vi "Draw Grid.vi"(8 "error in (no error)":errorcluster, 9 "color":u32(colorbox)=16777238, 11 "dialog info in":T1={"steering frame ref"=refnum, "active wheel indexes"=[], "FP Refs"={"VI Refnum"=refnum, "Menu Ref"=refnum, "Sub Panel"=refnum, "picture"=refnum, "Steering Type"=refnum, "zoom in"=refnum, "zoom out"=refnum, "zoom extents"=refnum, "Wheels"=refnum, "Add Wheel"=refnum, "Remove Wheel"=refnum, "Copy Wheel"=refnum, "Angle Units"=refnum}, "subpanel info"={"subpanel VI refs"=[], "subpanel types"=[], "main to subpanel command events"=[]}, "picture dragging state"={"dragging"=FALSE, "wheel index"=-1, "dragging mode"=enum."translate", "wheel start position"={"x"=0.0, "y"=0.0, "theta"=0.0}, "relative mouse position"={"x"=0.0, "y"=0.0}, "relative mouse init angle (rad)"=0.0}, "picture size (pixels)"={"Width"=500, "Height"=500}, "picture grid"=bytes[0], "click zones group"={"click zones array"=[], "num click zones"=0}, "draw options"={"draw wheel states?"=FALSE, "highlight wheel index"=-1, "pixels per unit"=10.0, "draw forward velocity?"=FALSE, "velocity scale"=1.0}}) -> (0 "error out":errorcluster, 3 "dialog info out":T1={"steering frame ref"=refnum, "active wheel indexes"=[], "FP Refs"={"VI Refnum"=refnum, "Menu Ref"=refnum, "Sub Panel"=refnum, "picture"=refnum, "Steering Type"=refnum, "zoom in"=refnum, "zoom out"=refnum, "zoom extents"=refnum, "Wheels"=refnum, "Add Wheel"=refnum, "Remove Wheel"=refnum, "Copy Wheel"=refnum, "Angle Units"=refnum}, "subpanel info"={"subpanel VI refs"=[], "subpanel types"=[], "main to subpanel command events"=[]}, "picture dragging state"={"dragging"=FALSE, "wheel index"=-1, "dragging mode"=enum."translate", "wheel start position"={"x"=0.0, "y"=0.0, "theta"=0.0}, "relative mouse position"={"x"=0.0, "y"=0.0}, "relative mouse init angle (rad)"=0.0}, "picture size (pixels)"={"Width"=500, "Height"=500}, "picture grid"=bytes[0], "click zones group"={"click zones array"=[], "num click zones"=0}, "draw options"={"draw wheel states?"=FALSE, "highlight wheel index"=-1, "pixels per unit"=10.0, "draw forward velocity?"=FALSE, "velocity scale"=1.0}})   [LabVIEW 2017, in "NI_Robotics_Configure Steering Frame.lvlib"]
uses:
  <vilib>/robotics/Dialog/Configure Steering Frame/NI_Robotics_Configure Steering Frame.lvlib
  <vilib>/robotics/Dialog/Configure Steering Frame/Dialog Info.ctl
  <vilib>/robotics/Steering/Steering Frame/NI_Robotics_Steering Frame.lvclass
  <vilib>/robotics/Dialog/Configure Steering Frame/FP Refs.ctl
  <vilib>/robotics/Dialog/Configure Steering Frame/Subpanel Info.ctl
  <vilib>/robotics/Dialog/Configure Steering Frame/Main to Subpanel Command Event.ctl
  <vilib>/robotics/Dialog/Configure Steering Frame/Main to Subpanel Command.ctl
  <vilib>/robotics/Dialog/Configure Steering Frame/Dragging State.ctl
  <vilib>/robotics/Dialog/Configure Steering Frame/Dragging Mode.ctl
  <vilib>/Utility/miscctls.llb/LVBoundsTypeDef.ctl
  <vilib>/robotics/Dialog/Configure Steering Frame/Click Zone.ctl
  <vilib>/robotics/Utilities/Visualization/Steering Visualization/Steering Picture/Draw Steering Frame Options.ctl
  <vilib>/robotics/Utilities/Visualization/Steering Visualization/Steering Picture/NI_Robotics_Steering Picture.lvlib
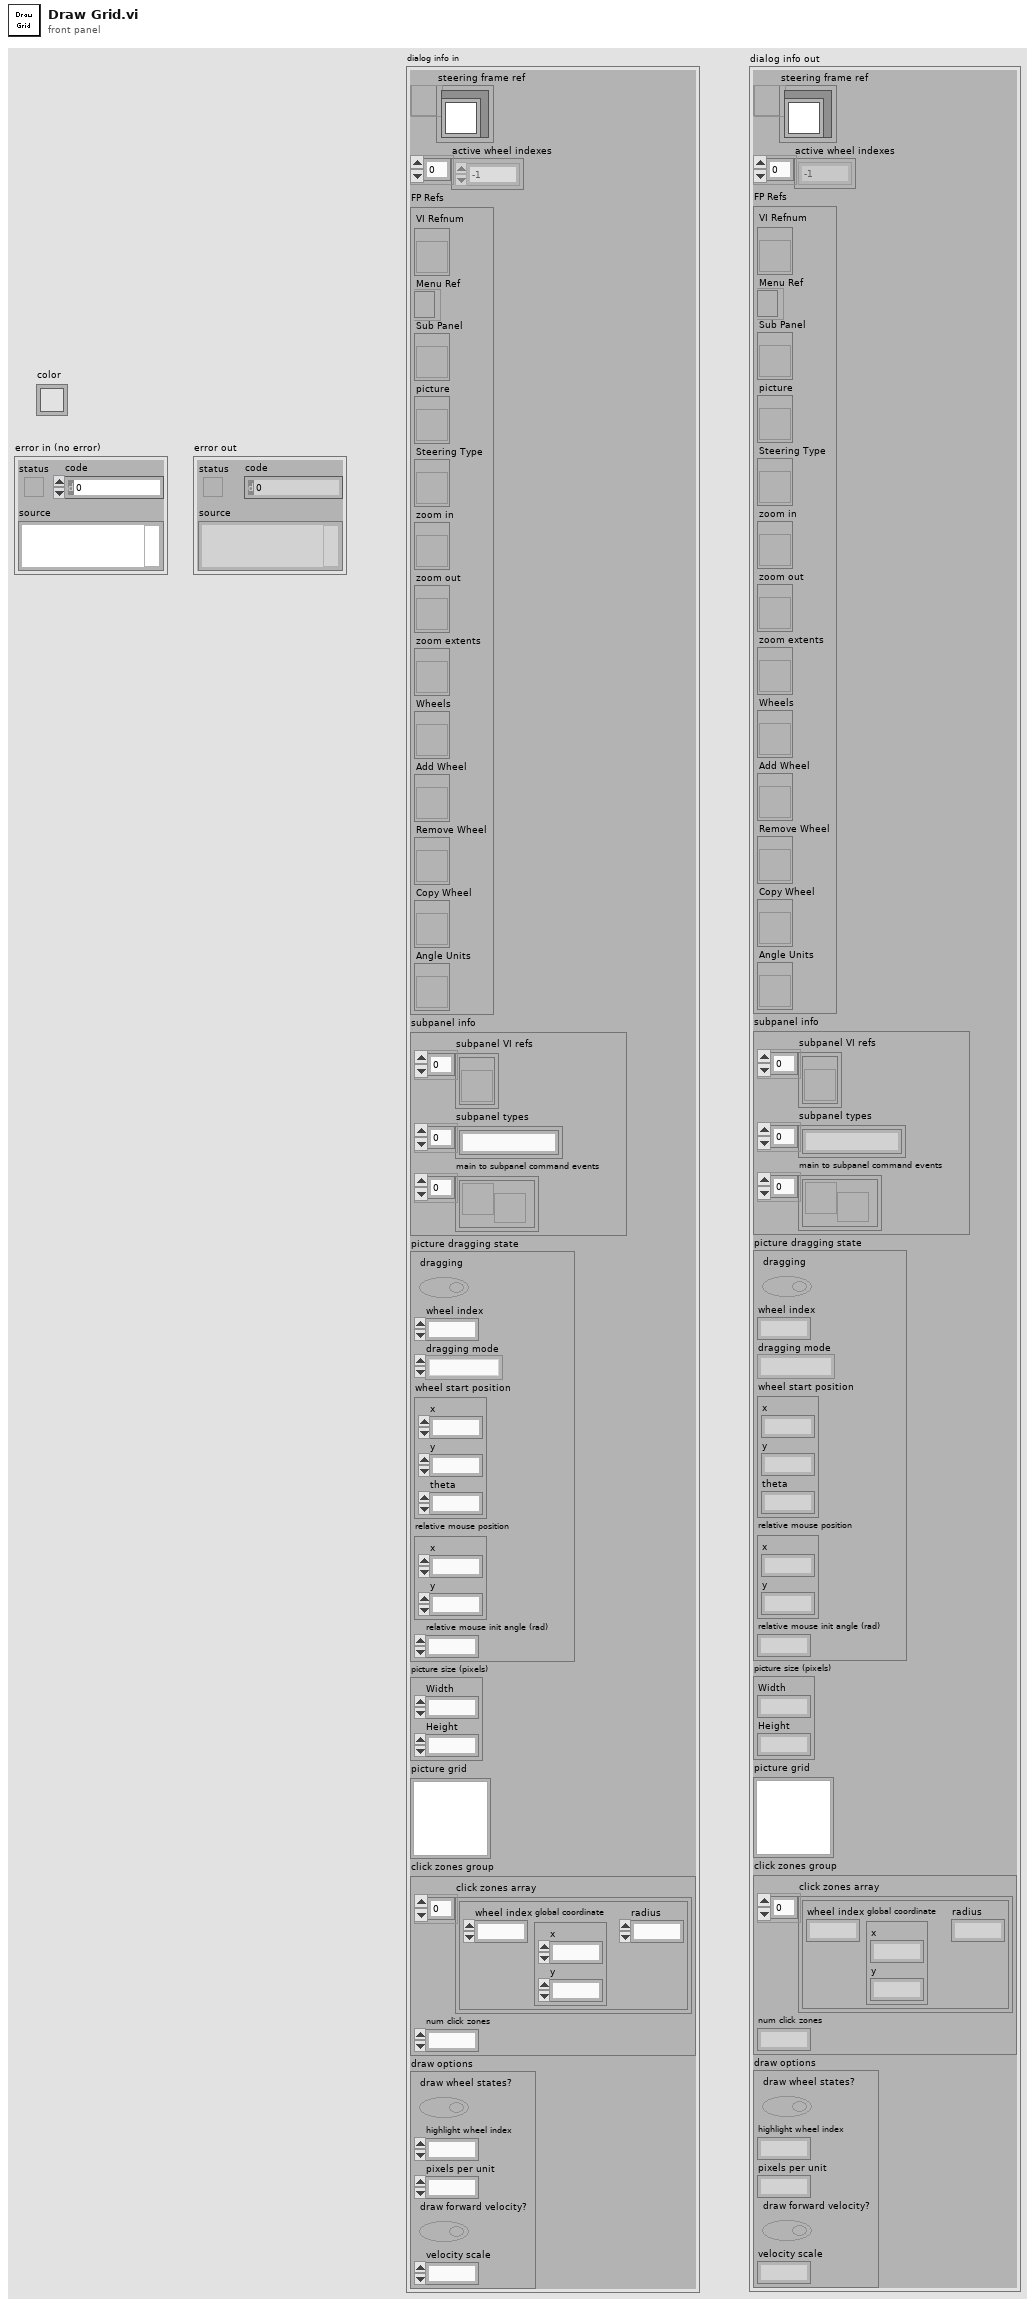
[diagram p1: front panel]
types:
  T1 = typedef "NI_Robotics_Configure Steering Frame.lvlib/Dialog Info.ctl" = cluster{"steering frame ref":refnum<data-value>, "active wheel indexes":i32[], "FP Refs":T2, "subpanel info":T3, "picture dragging state":T5, "picture size (pixels)":T7, "picture grid":picture, "click zones group":cluster{"click zones array":T8[], "num click zones":i32}, "draw options":T9}
  T2 = typedef "NI_Robotics_Configure Steering Frame.lvlib/FP Refs.ctl" = cluster{"VI Refnum":refnum<vi>, "Menu Ref":refnum<k9>, "Sub Panel":refnum<vi>, "picture":refnum<vi>, "Steering Type":refnum<vi>, "zoom in":refnum<vi>, "zoom out":refnum<vi>, "zoom extents":refnum<vi>, "Wheels":refnum<vi>, "Add Wheel":refnum<vi>, "Remove Wheel":refnum<vi>, "Copy Wheel":refnum<vi>, "Angle Units":refnum<vi>}
  T3 = typedef "NI_Robotics_Configure Steering Frame.lvlib/Subpanel Info.ctl" = cluster{"subpanel VI refs":refnum<vi>[], "subpanel types":string[], "main to subpanel command events":T4[]}
  T4 = typedef "NI_Robotics_Configure Steering Frame.lvlib/Main to Subpanel Command Event.ctl" = refnum<user-event>
  T5 = typedef "NI_Robotics_Configure Steering Frame.lvlib/Dragging State.ctl" = cluster{"dragging":bool, "wheel index":i32, "dragging mode":T6, "wheel start position":cluster{"x":dbl, "y":dbl, "theta":dbl}, "relative mouse position":cluster{"x":dbl, "y":dbl}, "relative mouse init angle (rad)":dbl}
  T6 = typedef "NI_Robotics_Configure Steering Frame.lvlib/Dragging Mode.ctl" = enum16{"translate", "rotate"}
  T7 = typedef "LVBoundsTypeDef.ctl" = cluster{"Width":u32, "Height":u32}
  T8 = typedef "NI_Robotics_Configure Steering Frame.lvlib/Click Zone.ctl" = cluster{"wheel index":i32, "global coordinate":cluster{"x":dbl, "y":dbl}, "radius":dbl}
  T9 = typedef "NI_Robotics_Steering Picture.lvlib/Draw Steering Frame Options.ctl" = cluster{"draw wheel states?":bool, "highlight wheel index":i32, "pixels per unit":dbl, "draw forward velocity?":bool, "velocity scale":dbl}
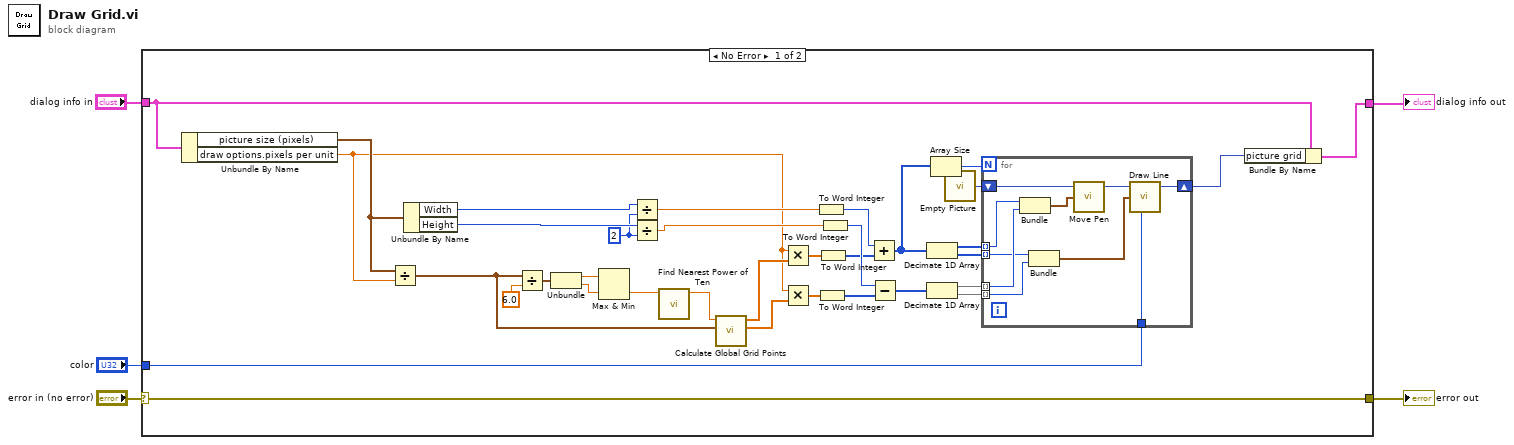
[diagram p0: block diagram]
diagram:
  n1 = case shown="No Error" "error in (no error)" {
    selector: "error in (no error)" -> [w40 w52]
    tunnel: [w40 w52] -> w4
    tunnel: "color" -> [w38 _]
    tunnel: "dialog info in" -> [w9 w51]
    tunnel: [w37 w51] -> w1
    frame No Error {
      w16 = u32 2 ("y")
      n2 = Unbundle By Name(w9) -> ("picture size (pixels)"=w10:T7, "draw options.pixels per unit"=w8:dbl)
      n3 = Divide(x=w10, y=w8) -> (x/y=w31:cluster{"Width":dbl, "Height":dbl})
      n4 = Unbundle By Name(w10) -> ("Width"=w15:u32, "Height"=w18:u32)
      n5 = Divide(x=w31, y=6.0) -> (x/y=w35:cluster{"Width":dbl, "Height":dbl})
      n6 = Unbundle(w35) -> ("Width"=w34:dbl, "Height"=w33:dbl)
      n7 = Max & Min(x=w34, y=w33) -> (min(x,y)=w32:dbl)  [unwired: 1 out]
      n8 = Divide(x=w15, y=w16) -> (x/y=w14:dbl)
      n9 = Divide(x=w18, y=w16) -> (x/y=w17:dbl)
      n10 = call <vilib>:"Find Nearest Power of Ten.vi"("n"=w32) -> ("nearest power of ten"=w6:dbl)  [unwired: 10 in]
      n11 = call <vilib>:"Calculate Global Grid Points.vi"("pictures size (units)"=w31, "grid spacing"=w6) -> ("y"=w29:dbl[], "x"=w30:dbl[])  [unwired: 8 in]
      n12 = Multiply(x=w8, y=w30) -> (x*y=w25:dbl[])
      n13 = Multiply(x=w8, y=w29) -> (x*y=w28:dbl[])
      n14 = To Word Integer(number=w14) -> (16bit integer=w11:i16)
      n15 = To Word Integer(number=w28) -> (16bit integer=w26:i16[])
      n16 = To Word Integer(number=w25) -> (16bit integer=w13:i16[])
      n17 = To Word Integer(number=w17) -> (16bit integer=w27:i16)
      n18 = Add(x=w11, y=w13) -> (x+y=w12:i16[])
      n19 = Subtract(x=w27, y=w26) -> (x-y=w24:i16[])
      n20 = Decimate 1D Array(w12) -> (w22:i16[], w21:i16[])
      n21 = Decimate 1D Array(w24) -> (w20:i16[], w19:i16[])
      n22 = Array Size(array=w12) -> (size(s)=w23:i32)
      n23 = call "Empty Picture"() -> ("empty picture"=w7:picture)
      n24 = for {
        N: w23 -> [_]
        shift-right: [w48] -> w39
        shift-left: w7 -> [w50]
        tunnel: w22 -> [w47] mode=indexing
        tunnel: w21 -> [w44] mode=indexing
        tunnel: w20 -> [w46] mode=indexing
        tunnel: w19 -> [w43] mode=indexing
        tunnel: w38 -> [w41]
        n25 = Bundle(w47, w46) -> (w45:cluster{i16, i16})  [unwired: 1 in]
        n26 = Bundle(w44, w43) -> (w42:cluster{i16, i16})  [unwired: 1 in]
        n27 = call <vilib>:"Move Pen.vi"("new position"=w45, "picture"=w50) -> ("new picture"=w49:picture)  [unwired: 3 in]
        n28 = call <vilib>:"Draw Line.vi"("picture"=w49, "end point"=w42, "color(black)"=w41) -> ("new picture"=w48:picture)  [unwired: 6 in]
      }
      n29 = Bundle By Name(cluster=w9, "picture grid"=w39) -> (w37:T1)
    }
    frame Error {
    }
  }
  "error out" <- w4
  "dialog info out" <- w1
